vi "Read Set.vi"(0 "VISA resource name":refnum<visa-resource-name>, 11 "error in (no error)":errorcluster) -> (1 "Local Lockout":u32(ring) items=["Off", "On"], 2 "ATTN":u32(ring) items=["Off", "On"], 3 "Run/Stop":u32(ring)=1 items=["Stop", "Run"], 4 "VISA resource name out":refnum<visa-resource-name>, 5 "Wavelength (nnnn)":dbl[unit], 6 "AVG":u32(ring) items=["Slow", "Medium", "Fast"], 9 "Range (1:8)":u32(ring) items=["Auto", "Lowest", "2", "3", "4", "5", "6", "7", "Highest"], 10 "Units":u32(ring)=1 items=["W"=1, "dB"=2, "dBm"=3, "REL"=4], 12 "Backlight":u32(ring) items=["Off", "Low", "High"], 13 "Beeper":u32(ring) items=["Off", "On"], 14 "Zero":u32(ring) items=["Off", "On"], 15 "error out":errorcluster)   [LabVIEW 2013]
doc: "Reads 1830-C options in succession and outputs their values.\n\nNote: Cannot tell if AutoRange is active."
uses:
  <vilib>/Utility/error.llb/DialogType.ctl
  Newport 1830-C.lvlib
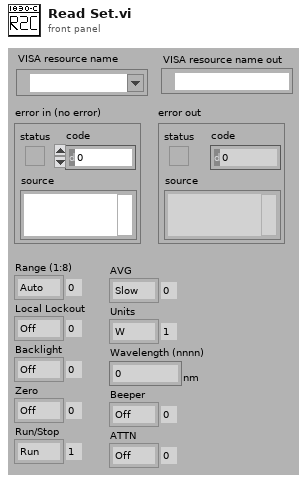
[diagram p1: front panel]
types:
  T1 = typedef "DialogType.ctl" = u16
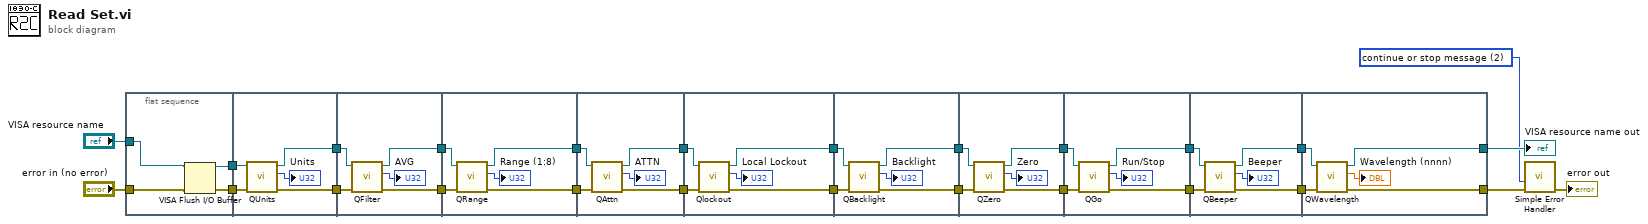
[diagram p0: block diagram]
diagram:
  w2 = T1 2 items=["no dialog", "OK message", "continue or stop message", "OK message + warnings", "continue/stop + warnings"] ("type of dialog (OK msg:1)")
  n1 = flat-sequence {
    tunnel: [w30] -> w7
    tunnel: "VISA resource name" -> [w27]
    tunnel: "error in (no error)" -> [w28]
    tunnel: [w29] -> w1
    tunnel: [w35] -> w26
    tunnel: [w32] -> w16
    tunnel: w7 -> [w34]
    tunnel: w1 -> [w33]
    tunnel: w26 -> [w40]
    tunnel: [w39] -> w25
    tunnel: w16 -> [w38]
    tunnel: [w37] -> w15
    tunnel: w25 -> [w45]
    tunnel: [w44] -> w24
    tunnel: w15 -> [w43]
    tunnel: [w42] -> w14
    tunnel: w24 -> [w50]
    tunnel: [w49] -> w23
    tunnel: w14 -> [w48]
    tunnel: [w47] -> w13
    tunnel: w23 -> [w55]
    tunnel: [w54] -> w22
    tunnel: w13 -> [w53]
    tunnel: [w52] -> w12
    tunnel: w22 -> [w60]
    tunnel: [w59] -> w21
    tunnel: w12 -> [w58]
    tunnel: [w57] -> w11
    tunnel: w21 -> [w65]
    tunnel: [w64] -> w20
    tunnel: w11 -> [w63]
    tunnel: [w62] -> w10
    tunnel: w20 -> [w70]
    tunnel: [w69] -> w19
    tunnel: w10 -> [w68]
    tunnel: [w67] -> w9
    tunnel: w19 -> [w75]
    tunnel: [w74] -> w18
    tunnel: w9 -> [w73]
    tunnel: [w72] -> w8
    tunnel: w18 -> [w80]
    tunnel: [w79] -> w17
    tunnel: w8 -> [w78]
    tunnel: [w77] -> w4
    frame #0 {
      n2 = VISA Flush I/O Buffer(VISA resource name=w27, error in (no error)=w28) -> (VISA resource name out=w30:refnum<visa-resource-name>, error out=w29:errorcluster)  [unwired: 1 in]
    }
    frame #1 {
      n3 = call "QUnits.vi"("error in (no error)"=w33, "VISA resource name"=w34) -> ("error out"=w32:errorcluster, "Units"=→"Units":u32, "VISA resource name out"=w35:refnum<visa-resource-name>)  [unwired: 6 in, 1 out]
    }
    frame #2 {
      n4 = call "QFilter.vi"("error in (no error)"=w38, "VISA resource name"=w40) -> ("error out"=w37:errorcluster, "Filter State"=→"AVG":u32, "VISA resource name out"=w39:refnum<visa-resource-name>)  [unwired: 7 in]
    }
    frame #3 {
      n5 = call "QRange.vi"("error in (no error)"=w43, "VISA resource name"=w45) -> ("error out"=w42:errorcluster, "Range"=→"Range (1:8)":u32, "VISA resource name out"=w44:refnum<visa-resource-name>)  [unwired: 7 in]
    }
    frame #4 {
      n6 = call "QAttn.vi"("error in (no error)"=w48, "VISA resource name"=w50) -> ("error out"=w47:errorcluster, "Attn State"=→"ATTN":u32, "VISA resource name out"=w49:refnum<visa-resource-name>)  [unwired: 7 in]
    }
    frame #5 {
      n7 = call "Qlockout.vi"("error in (no error)"=w53, "VISA resource name"=w55) -> ("error out"=w52:errorcluster, "Lockout State"=→"Local Lockout":u32, "VISA resource name out"=w54:refnum<visa-resource-name>)  [unwired: 7 in]
    }
    frame #6 {
      n8 = call "QBacklight.vi"("error in (no error)"=w58, "VISA resource name"=w60) -> ("error out"=w57:errorcluster, "BKLT State"=→"Backlight":u32, "VISA resource name out"=w59:refnum<visa-resource-name>)  [unwired: 7 in]
    }
    frame #7 {
      n9 = call "QZero.vi"("error in (no error)"=w63, "VISA resource name"=w65) -> ("error out"=w62:errorcluster, "Zero State"=→"Zero":u32, "VISA resource name out"=w64:refnum<visa-resource-name>)  [unwired: 7 in]
    }
    frame #8 {
      n10 = call "QGo.vi"("error in (no error)"=w68, "VISA resource name"=w70) -> ("error out"=w67:errorcluster, "Go State"=→"Run/Stop":u32, "VISA resource name out"=w69:refnum<visa-resource-name>)  [unwired: 7 in]
    }
    frame #9 {
      n11 = call "QBeeper.vi"("error in (no error)"=w73, "VISA resource name"=w75) -> ("error out"=w72:errorcluster, "Beeper State"=→"Beeper":u32, "VISA resource name out"=w74:refnum<visa-resource-name>)  [unwired: 7 in]
    }
    frame #10 {
      n12 = call "QWavelength.vi"("error in (no error)"=w78, "VISA resource name"=w80) -> ("error out"=w77:errorcluster, "Wavelength"=→"Wavelength (nnnn)":dbl[unit], "VISA resource name out"=w79:refnum<visa-resource-name>)  [unwired: 7 in]
    }
  }
  n13 = call <vilib>:"Simple Error Handler.vi"("type of dialog (OK msg:1)"=w2, "error in (no error)"=w4) -> ("error out"=→"error out":errorcluster)  [unwired: 3 in, 4 out]
  "VISA resource name out" <- w17
